vi "Init Mock.vi"(8 "error in (no error)":errorcluster, 11 "Mock In":refnum<class "LMock Mock.lvclass">) -> (0 "error out":errorcluster, 3 "Mock Out":refnum<class "LMock Mock.lvclass">)   [LabVIEW 2020, in "LMock Mock.lvclass"]
uses:
  LMock Mock.lvclass
  Core/Expectation/Expectation.lvclass
  Core/VI Call/VI Call.lvclass
  LMock Mock.lvclass/LMock Mock.ctl
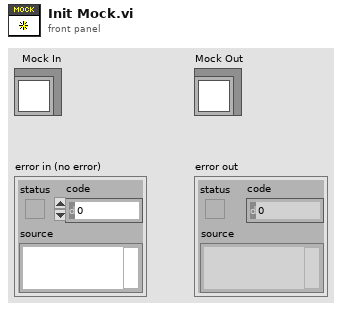
[diagram p1: front panel]
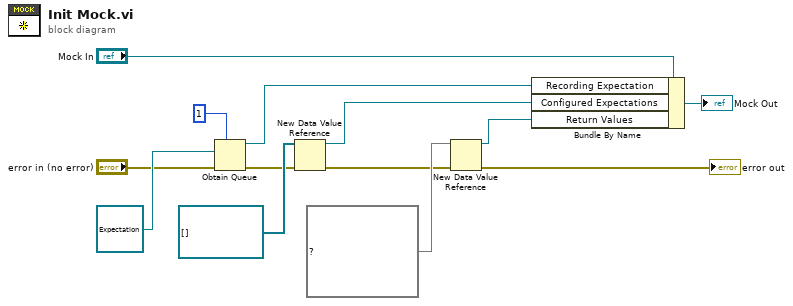
[diagram p0: block diagram]
diagram:
  n1 = Obtain Queue(max queue size (-1, unlimited)=1, element data type=refnum<class "Expectation.lvclass"> refnum ("Expectation.lvclass"), error in (no error)="error in (no error)") -> (queue out=w2:refnum<queue>, error out=w4:errorcluster)  [unwired: 2 in, 1 out]
  n2 = New Data Value Reference(data value=refnum<class "Expectation.lvclass">[] [] ("Array"), error in=w4) -> (data value reference=w10:refnum<data-value>, error out=w8:errorcluster)
  n3 = New Data Value Reference(data value=map{string, refnum<queue>} {} ("Return Values 2"), error in=w8) -> (data value reference=w6:refnum<data-value>, error out=→"error out":errorcluster)
  n4 = Bundle By Name(cluster="Mock In", "Recording Expectation"=w2, "Configured Expectations"=w10, "Return Values"=w6) -> (→"Mock Out":refnum<class "LMock Mock.lvclass">)
